vi "Check for End of Output Sweep.vi"(8 "error in (no error)":errorcluster, 10 "current generation level":dbl, 11 "measurement configuration":T1 {"acq sampling rate" format="%0.2f"; "master clock rate" format="%#_6pHz"; "frame clock rate" format="%#_6pHz"}) -> (0 "error out":errorcluster, 2 "generation level":dbl, 3 "sweep done":bool)   [LabVIEW 2021]
uses:
  Measurement Configuration.ctl
  shared/controls/digital audio protocol/data justification.ctl
  shared/controls/digital audio protocol/endianness.ctl
  shared/controls/digital audio protocol/digital edge.ctl
  shared/controls/digital audio protocol/logic level.ctl
  shared/controls/digital output level units.ctl
  shared/controls/weighting filter.ctl
  shared/controls/highpass filter.ctl
  shared/controls/lowpass filter.ctl
  shared/controls/sweep profile.ctl
  shared/controls/units - snr.ctl
  shared/controls/units - ratio.ctl
  shared/controls/regulation target.ctl
  shared/controls/regulation target value units.ctl
  shared/controls/audio controls.lvlib
  Stepped Frequency Sweep_Class D Amplifier.lvlib
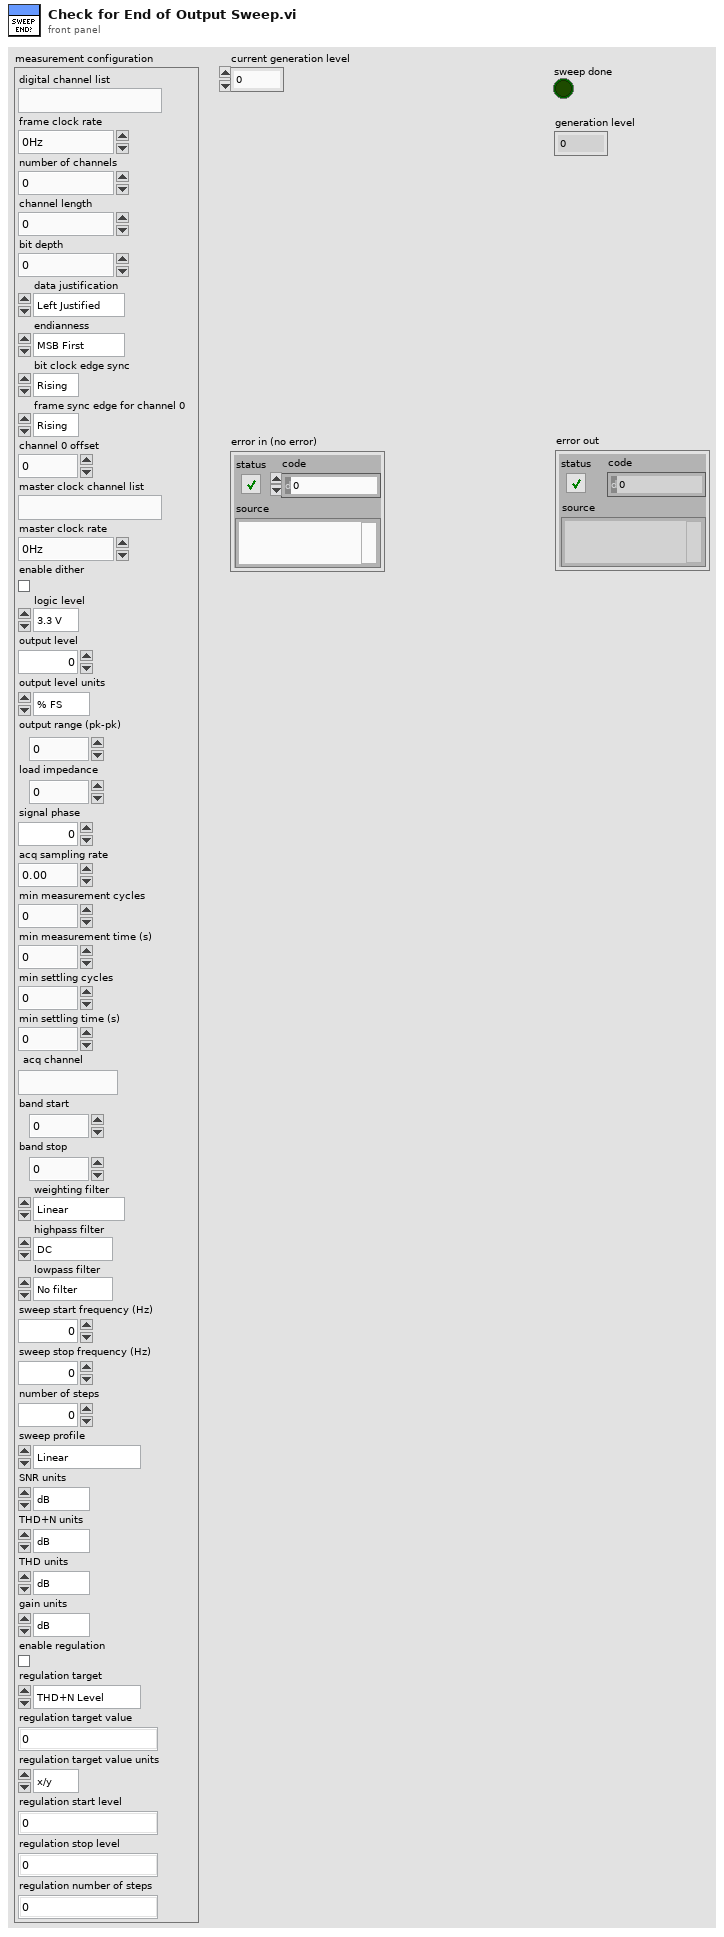
[diagram p1: front panel]
types:
  T1 = typedef "Stepped Frequency Sweep_Class D Amplifier.lvlib/Measurement Configuration.ctl" = cluster{"digital channel list":string, "frame clock rate":dbl, "number of channels":u32, "channel length":u32, "bit depth":u32, "data justification":T2, "endianness":T3, "bit clock edge sync":T4, "frame sync edge for channel 0":T4, "channel 0 offset":u32, "master clock channel list":string, "master clock rate":dbl, "enable dither":bool, "logic level":T5, "output level":dbl, "output level units":T6, "output range (pk-pk)":dbl, "load impedance":dbl, "signal phase":dbl, "acq sampling rate":dbl, "min measurement cycles":u32, "min measurement time (s)":dbl, "min settling cycles":u32, "min settling time (s)":dbl, "acq channel":string, "band start":dbl, "band stop":dbl, "weighting filter":T7, "highpass filter":T8, "lowpass filter":T9, "sweep start frequency (Hz)":dbl, "sweep stop frequency (Hz)":dbl, "number of steps":u32, "sweep profile":T10, "SNR units":T11, "THD+N units":T12, "THD units":T12, "gain units":T12, "enable regulation":bool, "regulation target":T13, "regulation target value":dbl, "regulation target value units":T14, "regulation start level":dbl, "regulation stop level":dbl, "regulation number of steps":u32}
  T2 = typedef "data justification.ctl" = enum32{"Left Justified", "Right Justified"}
  T3 = typedef "endianness.ctl" = enum32{"MSB First", "LSB First"}
  T4 = typedef "digital edge.ctl" = enum32{"Rising", "Falling"}
  T5 = typedef "logic level.ctl" = enum32{"3.3 V", "1.8 V", "1.2 V"}
  T6 = typedef "audio controls.lvlib/digital output level units.ctl" = enum32{"% FS", "dBFS"}
  T7 = typedef "weighting filter.ctl" = enum32{"Linear", "A-weighting", "B-weighting", "C-weighting"}
  T8 = typedef "highpass filter.ctl" = enum32{"DC", "AC"}
  T9 = typedef "lowpass filter.ctl" = enum32{"No filter", "AES17 20kHz", "AES17 40kHz"}
  T10 = typedef "audio controls.lvlib/sweep profile.ctl" = enum32{"Linear", "Logarithmic"}
  T11 = typedef "audio controls.lvlib/units - snr.ctl" = enum32{"dB", "x/y"}
  T12 = typedef "audio controls.lvlib/units - ratio.ctl" = enum32{"dB", "%", "x/y"}
  T13 = typedef "regulation target.ctl" = enum32{"THD+N Level", "THD+N Ratio", "RMS Level", "RMS Ratio", "Output Power"}
  T14 = typedef "regulation target value units.ctl" = enum32{"x/y", "%", "dB", "Vrms", "W"}
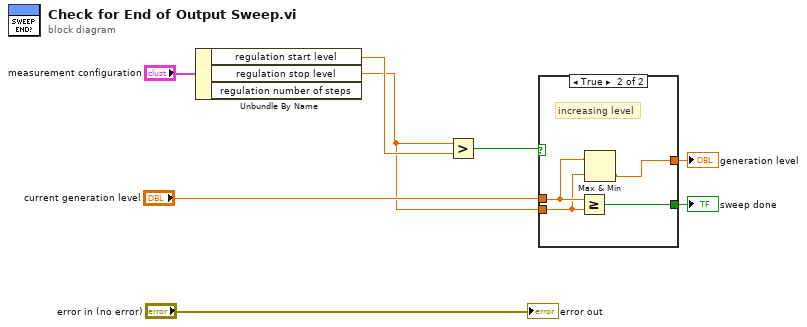
[diagram p0: block diagram]
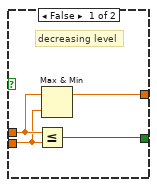
[diagram p2: hidden frame]
diagram:
  n1 = Unbundle By Name("measurement configuration") -> ("regulation start level"=w5:dbl, "regulation stop level"=w3:dbl)  [unwired: 1 out]
  n2 = Greater?(x=w3, y=w5) -> (0:w4:bool)
  n3 = case shown="True" w4 {
    tunnel: "current generation level" -> [w11 w15]
    tunnel: w3 -> [w10 w14]
    tunnel: [w12 w16] -> w2
    tunnel: [w9 w13] -> w1
    frame False {
      # "decreasing level"
      n4 = Less Or Equal?(x=w11, y=w10) -> (x <= y?=w12:bool)
      n5 = Max & Min(x=w11, y=w10) -> (max(x,y)=w9:dbl)  [unwired: 1 out]
    }
    frame True {
      # "increasing level"
      n6 = Greater Or Equal?(x=w15, y=w14) -> (x >= y?=w16:bool)
      n7 = Max & Min(x=w15, y=w14) -> (min(x,y)=w13:dbl)  [unwired: 1 out]
    }
  }
  "sweep done" <- w2
  "generation level" <- w1
  "error out" <- "error in (no error)"
